vi "saveAs.vi"(8 "error in (no error)":errorcluster, 11 "ScriptEditorV2 in":refnum<class "ScriptEditorV2.lvclass">) -> (0 "error out":errorcluster, 3 "ScriptEditorV2 out":refnum<class "ScriptEditorV2.lvclass">)   [LabVIEW 2011, in "Views.lvlib" / "ScriptEditor.lvlib" / "ScriptEditorV2.lvclass"]
uses:
  ScriptEditorV2.lvclass
  ScriptEditorV2.lvclass/ScriptEditorV2.ctl
  Tools/SettingsViewer/settingsViewer.lvclass
  Tools/Filing.lvlib
  Tools/Scripting/DataPointScript/DataPointScript.lvclass
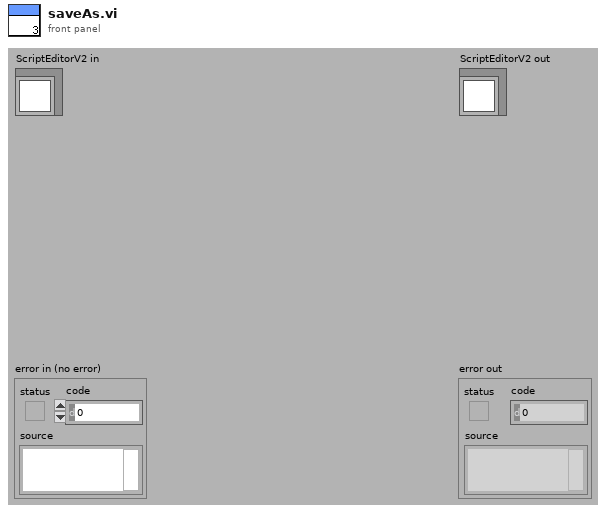
[diagram p1: front panel]
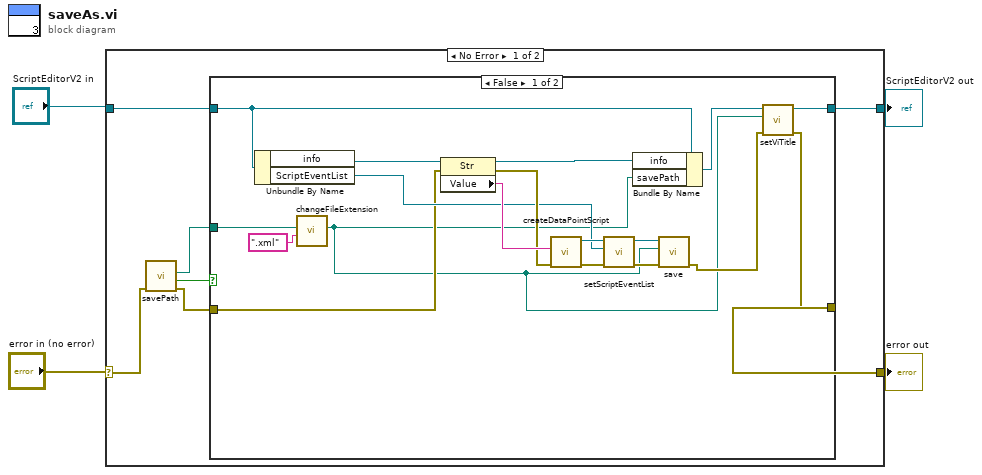
[diagram p0: block diagram]
diagram:
  n1 = case shown="No Error" "error in (no error)" {
    selector: "error in (no error)" -> [w11 w33]
    tunnel: [w5 w33] -> w3
    tunnel: [w6 w32] -> w1
    tunnel: "ScriptEditorV2 in" -> [w7 w32]
    frame No Error {
      n2 = call "savePath.vi"("error in (no error)"=w11) -> ("error out"=w8:errorcluster, "cancelled"=w10:bool, "Path out"=w9:path)  [unwired: 8 in]
      n3 = case shown="False" w10 {
        tunnel: w9 -> [w28 _]
        tunnel: w8 -> [w18 w30]
        tunnel: w7 -> [w17 w31]
        tunnel: [w15 w31] -> w6
        tunnel: [w13 w30] -> w5
        frame False {
          n4 = Unbundle By Name(w17) -> ("info"=w27:refnum<vi>, "ScriptEventList"=w21:refnum<class "ScriptEventList.lvclass">)
          n5 = call "changeFileExtension.vi"("extension"=".xml", "Path"=w28) -> ("Path out"=w12:path)  [unwired: 9 in]
          n6 = property class="Str"(reference=w27, error in=w18) -> (reference out=w24:refnum<vi>, error out=w25:errorcluster, "Value"=w26:string)
          n7 = call "createDataPointScript.vi"("error in (no error)"=w25, "script_comment"=w26) -> ("error out"=w23:errorcluster, "DataPointScript out"=w22:refnum<class "DataPointScript.lvclass">)  [unwired: 8 in]
          n8 = call "setScriptEventList.vi"("error in (no error)"=w23, "TScriptEventList"=w21, "DataPointScript.lvclass in"=w22) -> ("error out"=w20:errorcluster, "DataPointScript.lvclass out"=w19:refnum<class "DataPointScript.lvclass">)  [unwired: 7 in]
          n9 = Bundle By Name(cluster=w17, "info"=w24, "savePath"=w12) -> (w16:refnum<class "ScriptEditorV2.lvclass">)
          n10 = call "save.vi"("error in (no error)"=w20, "Path"=w12, "DataPointScript in"=w19) -> ("error out"=w14:errorcluster)  [unwired: 7 in, 1 out]
          n11 = call "setViTitle.vi"("error in (no error)"=w14, "Path"=w12, "ScriptEditorV2 in"=w16) -> ("error out"=w13:errorcluster, "ScriptEditorV2 out"=w15:refnum<class "ScriptEditorV2.lvclass">)  [unwired: 7 in]
        }
        frame True {
        }
      }
    }
    frame Error {
    }
  }
  "error out" <- w3
  "ScriptEditorV2 out" <- w1
